vi "smsFSM.vi"(0 "ATCMD":string) -> (1 "完成":bool, 2 "ATOK":string)   [LabVIEW 8.6]
doc: "使用该模板构建标准状态机设计模式。各状态执行代码并决定转移状态。将该设计模式与根据用户动作响应而执行代码的用户界面事件处理器模式相比较。同时将该设计模式与队列消息处理模式（各消息处理代码可排队0个或多个新消息）。"
uses:
  <vilib>/Instr/_visa.llb/Select Event Type.ctl
  smsFSM.ctl
  <vilib>/Instr/_visa.llb/VISA Configure Serial Port (Serial Instr).vi
panel:
  in  "波特率":u32 caption="波特率(9600)"
  in  "串行口":refnum<visa-resource-name>
  out "错误输出":errorcluster {"code" format="%.0x"}
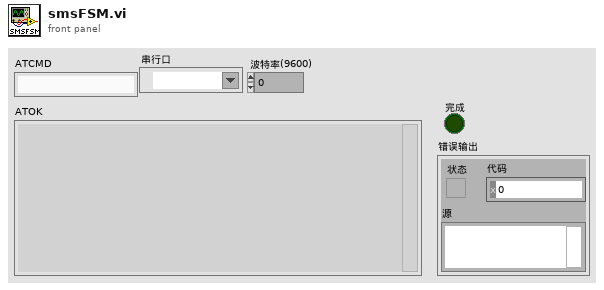
[diagram p1: front panel]
types:
  T1 = typedef "Select Event Type.ctl" = u32
  T2 = typedef "smsFSM.ctl" = enum16{"AT", "AT_OK", "AT_CMGS", "Stop"}
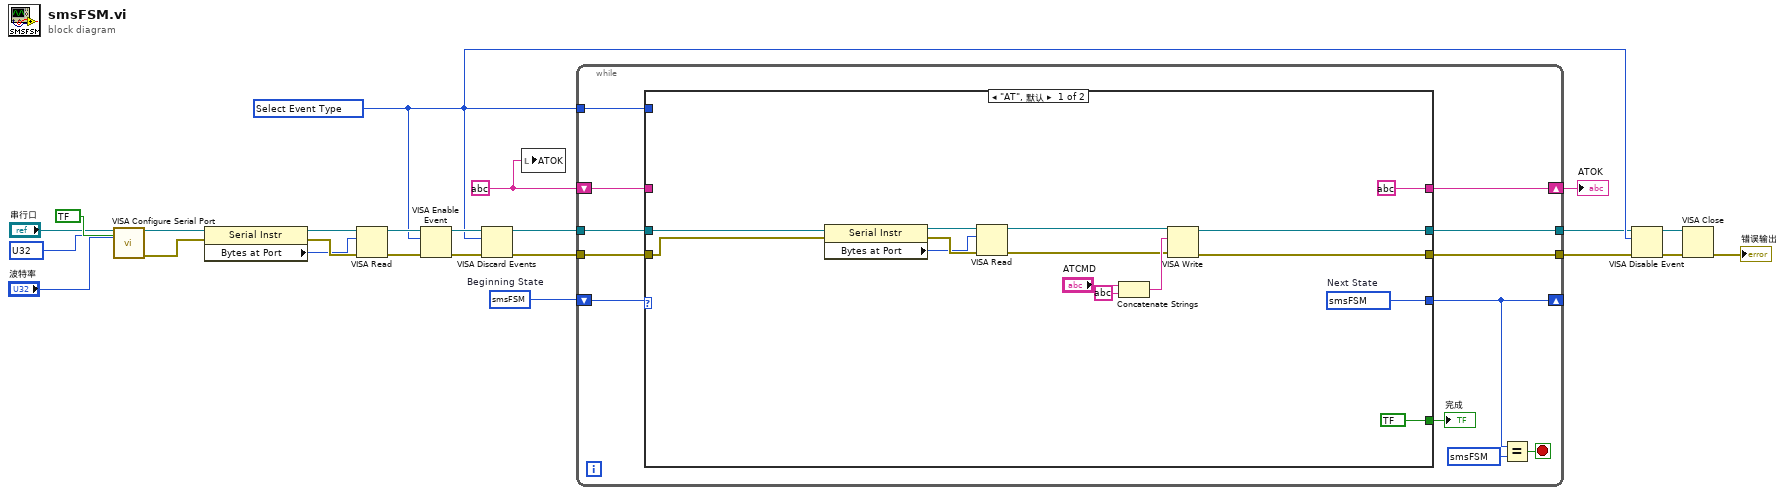
[diagram p0: block diagram]
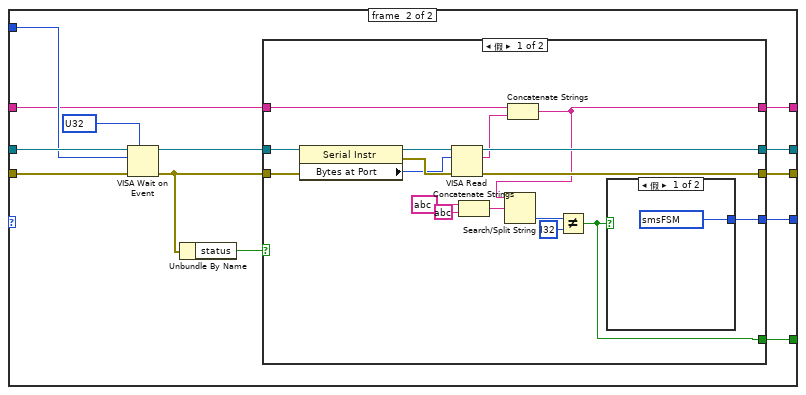
[diagram p2: hidden frame]
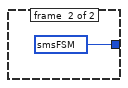
[diagram p3: hidden frame]
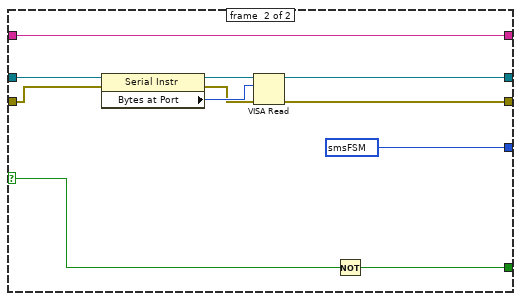
[diagram p4: hidden frame]
diagram:
  w15 = string ?
  w6 = T1 ? items=["ServiceRequest", "Trigger", "Clear", "VXI-Signal", "VXI/VME-Interrupt", "VXI/VME-Sysfail", "VXI/VME-Sysreset", "GPIB-CIC", "GPIB-Talk", "GPIB-Listen", "PXI-Interrupt", "AllEnabled", "Serial-Break", "Serial-TermChar", "Serial-CTS", "Serial-DSR", "Serial-DCD", "Serial-RI", "Serial-Character"] ("Event Type")
  w24 = T2 ?  # Beginning State
  n1 = call-poly "VISA Configure Serial Port"("VISA resource name"="串行口", "timeout (10sec)"=u32 ? ("超时"), "Enable Termination\nChar (T)"=bool ? ("Enable Termination Char (T)"), "baud rate (9600)"="波特率") -> ("VISA resource name out"=w10:refnum<visa-resource-name>, "error out"=w9:errorcluster)  [unwired: 4 in, 6 out]
  n2 = property class="Serial Instr"(reference=w10, error in=w9) -> (reference out=w13:refnum<visa-resource-name>, error out=w12:errorcluster, "Bytes at Port"=w11:u32)
  n3 = VISA Read(VISA resource name=w13, byte count=w11, error in (no error)=w12) -> (VISA resource name out=w8:refnum<visa-resource-name>, error out=w7:errorcluster)  [unwired: 2 out]
  n4 = VISA Enable Event(8:w7, 10:w6, 11:w8) -> (0:w20:errorcluster, 3:w21:refnum<visa-resource-name>)  [unwired: 1 out]
  n5 = VISA Discard Events(8:w20, 10:w6, 11:w21) -> (0:w16:errorcluster, 3:w17:refnum<visa-resource-name>)  [unwired: 1 out]
  n6 = local write "ATOK"(w15) -> ()
  n7 = while {
    shift-right: [w27] -> _
    shift-left: w24 -> [w34]
    tunnel: w17 -> [w33]
    tunnel: w16 -> [w32]
    tunnel: [w31] -> w5
    tunnel: [w30] -> w4
    tunnel: w6 -> [w29]
    shift-right: [w26] -> w14
    shift-left: w15 -> [w28]
    stop <- w36 stop-if-true
    n8 = case shown="\"AT\", 默认" w34 {
      tunnel: [w51 w55] -> w27
      tunnel: w33 -> [w40 w62]
      tunnel: w32 -> [w39 w61]
      tunnel: [w47 w60] -> w31
      tunnel: [w46 w57] -> w30
      tunnel: w29 -> [_ w59]
      tunnel: w28 -> [_ w58]
      tunnel: [string ? w56] -> w26
      tunnel: [bool ? w54] -> w25
      frame #0 {
        w51 = T2 ?  # Next State
        n9 = property class="Serial Instr"(reference=w40, error in=w39) -> (reference out=w43:refnum<visa-resource-name>, error out=w42:errorcluster, "Bytes at Port"=w41:u32)
        n10 = VISA Read(VISA resource name=w43, byte count=w41, error in (no error)=w42) -> (VISA resource name out=w38:refnum<visa-resource-name>, error out=w37:errorcluster)  [unwired: 2 out]
        n11 = Concatenate Strings("ATCMD", string ?) -> (w50:string)
        n12 = VISA Write(VISA resource name=w38, write buffer=w50, error in (no error)=w37) -> (VISA resource name out=w47:refnum<visa-resource-name>, error out=w46:errorcluster)  [unwired: 1 out]
      }
      frame #1 {
        n13 = VISA Wait on Event(7:u32 ? ("超时"), 8:w61, 10:w59, 11:w62) -> (0:w64:errorcluster, 3:w63:refnum<visa-resource-name>)  [unwired: 1 in, 2 out]
        n14 = Unbundle By Name(w64) -> ("status"=w53:bool)
        n15 = case shown="假" w53 {
          selector: w53 -> [_ w93]
          tunnel: w63 -> [w81 w87]
          tunnel: w64 -> [w80 w86]
          tunnel: [w79 w85] -> w60
          tunnel: [w78 w84] -> w57
          tunnel: w58 -> [w77 w92]
          tunnel: [w66 w92] -> w56
          tunnel: [w76 T2 ? ("Next State")] -> w55
          tunnel: [w67 w94] -> w54
          frame #0 {
            n16 = property class="Serial Instr"(reference=w81, error in=w80) -> (reference out=w75:refnum<visa-resource-name>, error out=w74:errorcluster, "Bytes at Port"=w73:u32)
            n17 = VISA Read(VISA resource name=w75, byte count=w73, error in (no error)=w74) -> (VISA resource name out=w79:refnum<visa-resource-name>, read buffer=w65:string, error out=w78:errorcluster)  [unwired: 1 out]
            n18 = Concatenate Strings(string ? ("搜索字符串/字符(-)"), string ?) -> (w68:string)
            n19 = Concatenate Strings(w77, w65) -> (w66:string)
            n20 = Search/Split String(string=w66, search string/char (-)=w68) -> (offset of match=w71:i32)  [unwired: 1 in, 2 out]
            n21 = Not Equal?(x=w71, y=i32 ?) -> (x != y?=w67:bool)
            n22 = case shown="假" w67 {
              tunnel: [T2 ? ("Next State") T2 ? ("Next State")] -> w76
              frame #0 {
              }
              frame #1 {
              }
            }
          }
          frame #1 {
            n23 = property class="Serial Instr"(reference=w87, error in=w86) -> (reference out=w88:refnum<visa-resource-name>, error out=w89:errorcluster, "Bytes at Port"=w90:u32)
            n24 = VISA Read(VISA resource name=w88, byte count=w90, error in (no error)=w89) -> (VISA resource name out=w85:refnum<visa-resource-name>, error out=w84:errorcluster)  [unwired: 2 out]
            n25 = Not(x=w93) -> (.not. x?=w94:bool)
          }
        }
      }
    }
    "完成" <- w25
    n26 = Equal?(x=w27, y=T2 ? ("States")) -> (x = y?=w36:bool)
  }
  "ATOK" <- w14
  n27 = VISA Disable Event(8:w4, 10:w6, 11:w5) -> (0:w18:errorcluster, 3:w19:refnum<visa-resource-name>)  [unwired: 1 out]
  n28 = VISA Close(VISA resource name=w19, error in (no error)=w18) -> (error out=→"错误输出":errorcluster)
